vi "CRYHardware.vi"(0 "Setup in":T6={"No.VI"=0, "Category"="", "StepName"="", "Seq setup flattened"="", "Comment"="", "Steps config."=[], "Jump config"=[], "Start"=0.0, "Increment"=0.0, "Name"="Pa", "Unit"="Pa", "Y data"=1, "Y prefix"="", "Y dB ref"=1.0, "Y unit"="", "Repeat State Array"=[]} {"Repeat State Array"."Start" format="%#_5g"; "Y dB ref" format="%.1f"; "Y data" items=["dB", "Lin"]; "Start" format="%#_5g"}, 5 "Data in":T4 {"Z data" items=["dB", "Lin"]; "X data" items=["dB", "Lin"]; "Y data" items=["dB", "Lin"]; "Z dB ref" format="%.1f"; "Z axis" items=["Log", "Lin"]; "X dB ref" format="%.1f"; "X axis" items=["Log", "Lin"]; "Y axis" items=["Log", "Lin"]; "Y dB ref" format="%.1f"; "Curve"."z" format="%.2f"; "Curve"."y" format="%.2f"; "Curve"."x" format="%.2f"}, 7 "Results in":T2 {"Margin" format="%.2f"}, 9 "Seq Setup in":string, 11 "Step name":string, 12 "Hardware in":string, 13 "Calibration in":string) -> (3 "Types Out":string[](array[string]), 4 "Inserted Names Out":string[](array[string]), 6 "Data out":T4 {"Z data" items=["dB", "Lin"]; "X data" items=["dB", "Lin"]; "Y data" items=["dB", "Lin"]; "Z dB ref" format="%.1f"; "Z axis" items=["Log", "Lin"]; "X dB ref" format="%.1f"; "X axis" items=["Log", "Lin"]; "Y axis" items=["Log", "Lin"]; "Y dB ref" format="%.1f"; "Curve"."z" format="%.2f"; "Curve"."y" format="%.2f"; "Curve"."x" format="%.2f"}, 8 "Results out":T2 {"Margin" format="%.2f"}, 10 "Wave out":T1[](array[typedef]) {"Y dB ref" format="%.1f"; "Y axis" items=["Log", "Lin"]; "Y data" items=["dB", "Lin"]; "X data" items=["dB", "Lin"]})   [LabVIEW 2013]
uses:
  Typedef Control/CRYData Cluster Array.ctl
  Typedef Control/CRYData Cluster.ctl
  Typedef Control/CRYResult Cluster Array.ctl
  Typedef Control/CRYResult Cluster.ctl
  Typedef Control/CRYStep.ctl
  Typedef Control/CRYWaveform Cluster.ctl
  CRYHardware Global.vi
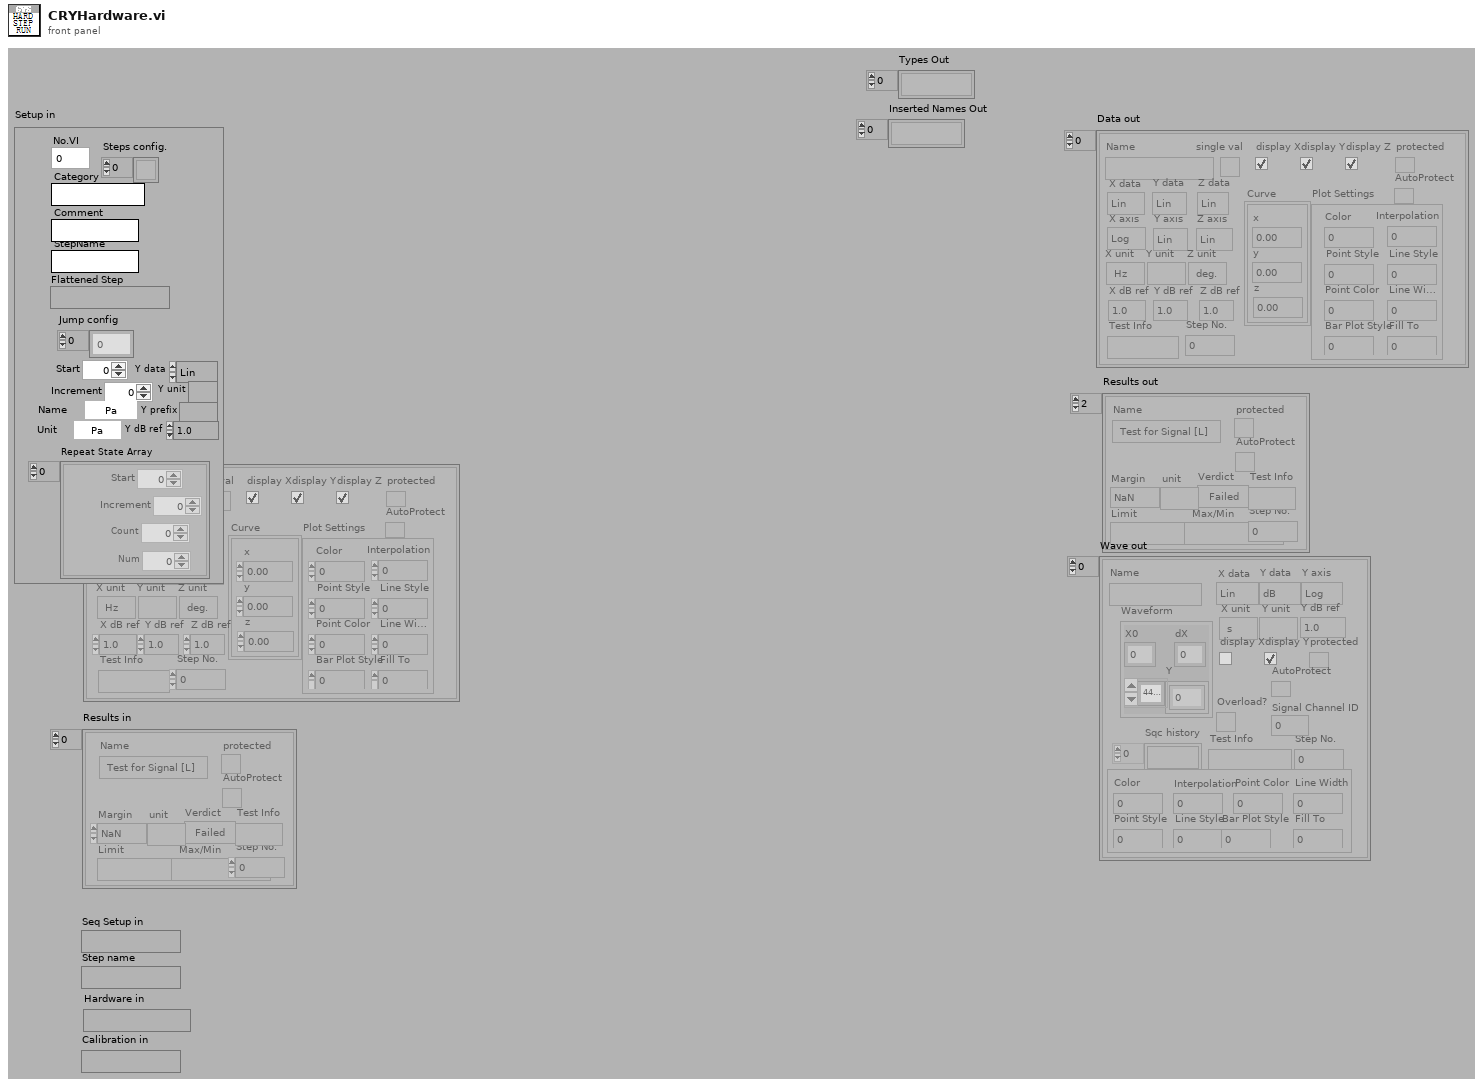
[diagram p1: front panel]
types:
  T1 = typedef "CRYWaveform Cluster.ctl" = cluster{"Waveform":cluster{"X0":dbl, "dX":dbl, "Y":sgl[]}, "X data":u16, "Y data":u16, "Y axis":u16, "X unit":string, "Y unit":string, "Y dB ref":dbl, "display Y":bool, "display X":bool, "Overload?":bool, "Test Info":string, "Step No.":i32, "Name":string, "protected":bool, "Sqc history":string[], "Signal Channel ID":i32, "Plot Settings":cluster{"Color":u32, "Interpolation":u8, "Point Style":u8, "Line Style":u8, "Point Color":u32, "Line Width":u8, "Bar Plot Style":u8, "Fill To":i16}, "AutoProtect":bool}
  T2 = typedef "CRYResult Cluster Array.ctl" = T3[]
  T3 = typedef "CRYResult Cluster.ctl" = cluster{"Name":string, "Margin":dbl, "unit":string, "Verdict":bool, "Limit":string, "Max/Min":string, "protected":bool, "Step No.":i32, "Test Info":string, "AutoProtect":bool}
  T4 = typedef "CRYData Cluster Array.ctl" = T5[]
  T5 = typedef "CRYData Cluster.ctl" = cluster{"Name":string, "Curve":cluster{"x":dbl, "y":dbl, "z":dbl}[], "X data":u16, "Y data":u16, "Z data":u16, "X axis":u16, "Y axis":u16, "Z axis":u16, "X unit":string, "Y unit":string, "Z unit":string, "X dB ref":dbl, "Y dB ref":dbl, "Z dB ref":dbl, "single val":bool, "protected":bool, "display X":bool, "display Y":bool, "display Z":bool, "Test Info":string, "Step No.":i32, "Plot Settings":cluster{"Color":u32, "Interpolation":u8, "Point Style":u8, "Line Style":u8, "Point Color":u32, "Line Width":u8, "Bar Plot Style":u8, "Fill To":i16}, "AutoProtect":bool}
  T6 = typedef "CRYStep.ctl" = cluster{"No.VI":i32, "Category":string, "StepName":string, "Seq setup flattened":string, "Comment":string, "Steps config.":bool[], "Jump config":i32[], "Start":dbl, "Increment":dbl, "Name":string, "Unit":string, "Y data":u16, "Y prefix":string, "Y dB ref":dbl, "Y unit":string, "Repeat State Array":cluster{"Start":dbl, "Increment":dbl, "Count":i32, "Num":i32}[]}
  T7 = typedef "CRY6175Hardware.ctl" = cluster{"Tab Value":u16, "Help":string, "In Channel 1":u16, "In Channel 2":u16, "In Gain 1":i32, "In Gain 2":i32, "Mic Volt":i32, "Mic Resis":i32, "Out Channel":u16, "OUT_Impedance 1":u16, "OUT_Impedance 2":u16, "IN_Channel 1 Old":u16}
  T8 = enum16{"OK", "Yes", "YesNo", "YesNoCancel", "ReplaceAppend"}
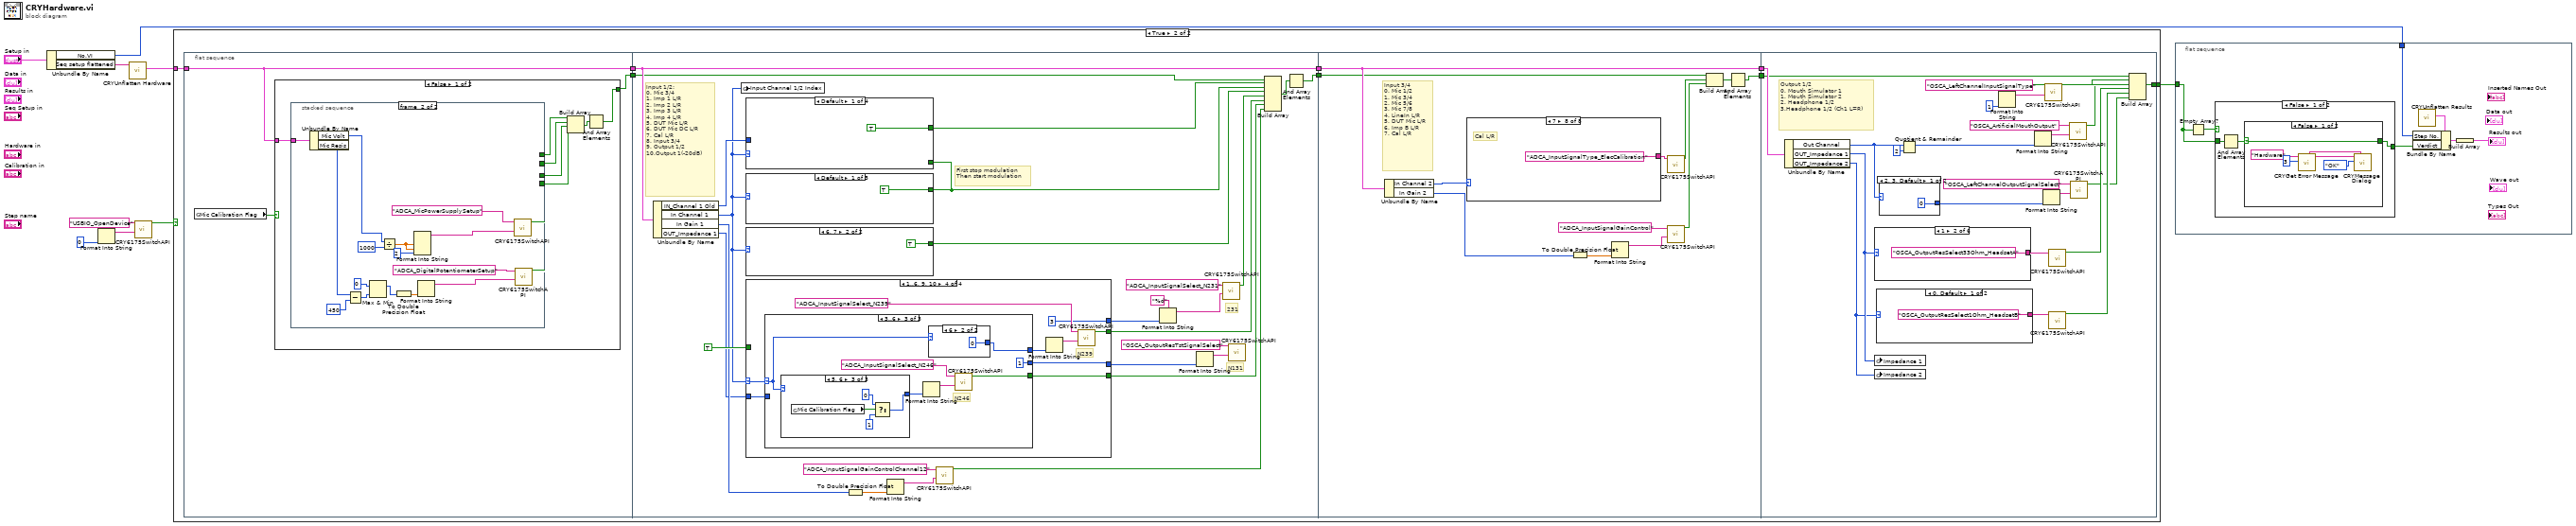
[diagram p0: block diagram]
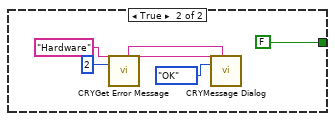
[diagram p3: hidden frame]
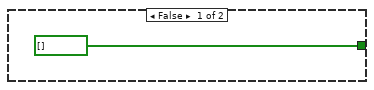
[diagram p4: hidden frame]
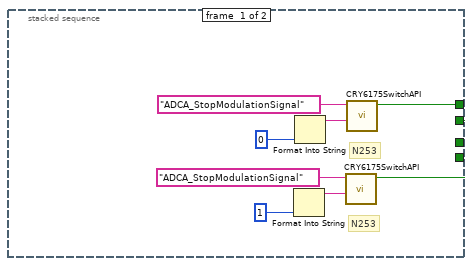
[diagram p5: hidden frame]
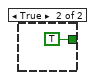
[diagram p6: hidden frame]
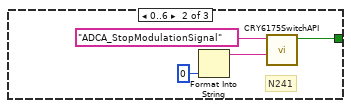
[diagram p7: hidden frame]
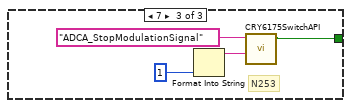
[diagram p8: hidden frame]
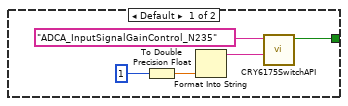
[diagram p9: hidden frame]
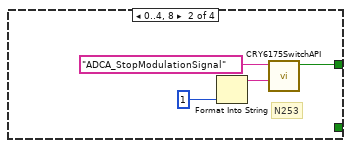
[diagram p10: hidden frame]
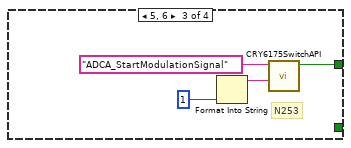
[diagram p11: hidden frame]
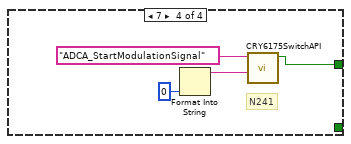
[diagram p12: hidden frame]
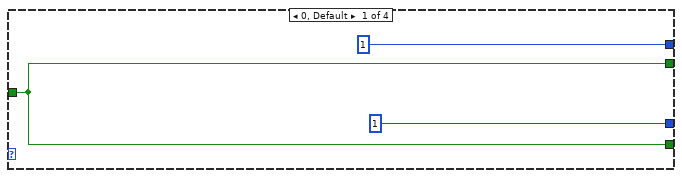
[diagram p13: hidden frame]
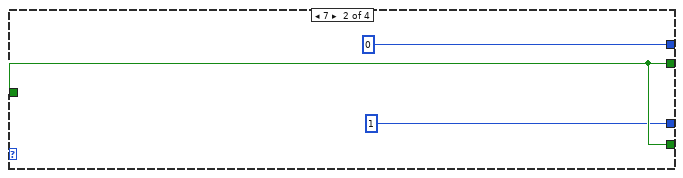
[diagram p14: hidden frame]
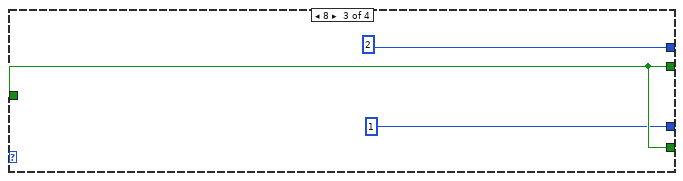
[diagram p15: hidden frame]
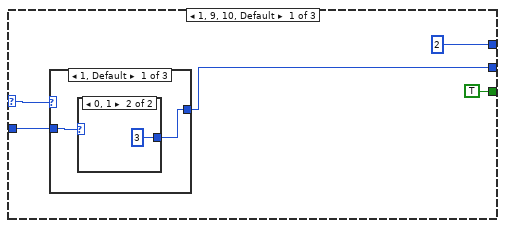
[diagram p16: hidden frame]
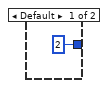
[diagram p17: hidden frame]
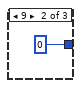
[diagram p18: hidden frame]
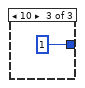
[diagram p19: hidden frame]
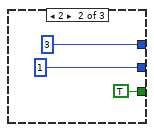
[diagram p20: hidden frame]
diagram:
  n1 = Unbundle By Name("Setup in") -> ("No.VI"=w2:i32, "Seq setup flattened"=w8:string)
  n2 = Format Into String(0) -> (resulting string=w3:string)  [unwired: 3 in, 1 out]
  n3 = call "CRYUnflatten Hardware.vi"("Unflatten Hardware#"=w8) -> ("Hardware"=w6:T7)  [unwired: 8 in, 2 out]
  n4 = call "CRY6175SwitchAPI.vi"("Parameter"=w3, "Function Name"="USBIO_OpenDevice") -> ("bResult"=w1:bool)  [unwired: 9 in]
  n5 = case shown="True" w1 {
    tunnel: w6 -> [_ w12]
    tunnel: [bool[] [] w14] -> w7
    frame False {
    }
    frame True {
      n6 = flat-sequence {
        tunnel: [w20] -> w13
        tunnel: w12 -> [w20]
        tunnel: [w21] -> w11
        tunnel: [w56] -> w18
        tunnel: [w62] -> w16
        tunnel: w13 -> [w56]
        tunnel: w11 -> [w55]
        tunnel: w18 -> [w162]
        tunnel: [w162] -> w17
        tunnel: w16 -> [w161]
        tunnel: [w157] -> w15
        tunnel: w17 -> [w198]
        tunnel: w15 -> [w192]
        tunnel: [w188] -> w14
        frame #0 {
          n7 = global read "CRYHardware Global.vi" "Mic Calibration Flag"() -> (w19:bool)
          n8 = case shown="False" w19 {
            tunnel: [w22 TRUE] -> w21
            tunnel: w20 -> [w23 _]
            frame False {
              n9 = stacked-sequence {
                tunnel: [w29 _] -> w25
                tunnel: [w30 _] -> w26
                tunnel: w23 -> [_ w39]
                tunnel: [_ w38] -> w28
                tunnel: [_ w37] -> w27
                frame #0 {
                  # "N253"
                  # "N253"
                  n10 = Format Into String(u16 1 ("input 1")) -> (resulting string=w32:string)  [unwired: 3 in, 1 out]
                  n11 = Format Into String(u16 0 ("input 1")) -> (resulting string=w35:string)  [unwired: 3 in, 1 out]
                  n12 = call "CRY6175SwitchAPI.vi"("Parameter"=w32, "Function Name"="ADCA_StopModulationSignal") -> ("bResult"=w30:bool)  [unwired: 9 in]
                  n13 = call "CRY6175SwitchAPI.vi"("Parameter"=w35, "Function Name"="ADCA_StopModulationSignal") -> ("bResult"=w29:bool)  [unwired: 9 in]
                }
                frame #1 {
                  n14 = Unbundle By Name(w39) -> ("Mic Volt"=w52:i32, "Mic Resis"=w53:i32)
                  n15 = Subtract(x=w53, y=450) -> (x-y=w49:i32)
                  n16 = Max & Min(x=0 ("y"), y=w49) -> (max(x,y)=w51:i32)  [unwired: 1 out]
                  n17 = Divide(x=w52, y=1000) -> (x/y=w44:dbl)
                  n18 = To Double Precision Float(number=w51) -> (double precision float=w41:dbl)
                  n19 = Format Into String(w44, w44, 2 ("input 3")) -> (resulting string=w42:string)  [unwired: 3 in, 1 out]
                  n20 = Format Into String(w41) -> (resulting string=w40:string)  [unwired: 3 in, 1 out]
                  n21 = call "CRY6175SwitchAPI.vi"("Parameter"=w42, "Function Name"="ADCA_MicPowerSupplySetup") -> ("bResult"=w37:bool)  [unwired: 9 in]
                  n22 = call "CRY6175SwitchAPI.vi"("Parameter"=w40, "Function Name"="ADCA_DigitalPotentiometerSetup") -> ("bResult"=w38:bool)  [unwired: 9 in]
                }
              }
              n23 = Build Array(w25, w26, w27, w28) -> (w24:bool[])
              n24 = And Array Elements(Boolean array=w24) -> (logical AND=w22:bool)
            }
            frame True {
            }
          }
        }
        frame #1 {
          # "First stop modulation\nThen start modulation"
          # "Input 1/2:\n0. Mic 3/4\n1. Imp 1 L/R\n2. Imp 2 L/R\n3. Imp 3 L/R\n4. Imp 4 L/R\n5. DUT Mic L/R\n6. DUT Mic DC L/R\n7. Cal L/R\n8. Input 3/4\n9. Output 1/2 \n10.Output 1(-20dB)"
          # "N131"
          # "231"
          n25 = Unbundle By Name(w56) -> ("IN_Channel 1 Old"=w61:u16, "In Channel 1"=w57:u16, "In Gain 1"=w60:i32, "OUT_Impedance 1"=w58:u16)
          n26 = global write "CRYHardware Global.vi" "Input Channel 1/2 Index"(w57) -> ()
          n27 = case shown="Default" w57 {
            tunnel: [TRUE ("bResult") w82 w86] -> w59
            frame Default {
            }
            frame 0..6 {
              # "N241"
              n28 = Format Into String(u16 0 ("input 1")) -> (resulting string=w85:string)  [unwired: 3 in, 1 out]
              n29 = call "CRY6175SwitchAPI.vi"("Parameter"=w85, "Function Name"="ADCA_StopModulationSignal") -> ("bResult"=w82:bool)  [unwired: 9 in]
            }
            frame 7 {
              # "N253"
              n30 = Format Into String(u16 1 ("input 1")) -> (resulting string=w88:string)  [unwired: 3 in, 1 out]
              n31 = call "CRY6175SwitchAPI.vi"("Parameter"=w88, "Function Name"="ADCA_StopModulationSignal") -> ("bResult"=w86:bool)  [unwired: 9 in]
            }
          }
          n32 = case shown="Default" w57 {
            tunnel: [TRUE ("bResult") w99 w104 w105] -> w65
            tunnel: w61 -> [_ _ _ _]
            tunnel: w59 -> [_ _ _ _]
            frame Default {
            }
            frame 0..4, 8 {
              # "N253"
              n33 = Format Into String(u16 1 ("input 1")) -> (resulting string=w98:string)  [unwired: 3 in, 1 out]
              n34 = call "CRY6175SwitchAPI.vi"("Parameter"=w98, "Function Name"="ADCA_StopModulationSignal") -> ("bResult"=w99:bool)  [unwired: 9 in]
            }
            frame 5, 6 {
              # "N253"
              n35 = Format Into String(u16 1 ("input 1")) -> (resulting string=w102:string)  [unwired: 3 in, 1 out]
              n36 = call "CRY6175SwitchAPI.vi"("Parameter"=w102, "Function Name"="ADCA_StartModulationSignal") -> ("bResult"=w104:bool)  [unwired: 9 in]
            }
            frame 7 {
              # "N241"
              n37 = Format Into String(u16 0 ("input 1")) -> (resulting string=w106:string)  [unwired: 3 in, 1 out]
              n38 = call "CRY6175SwitchAPI.vi"("Parameter"=w106, "Function Name"="ADCA_StartModulationSignal") -> ("bResult"=w105:bool)  [unwired: 9 in]
            }
          }
          n39 = case shown="6, 7" w57 {
            tunnel: [w90 TRUE ("bResult")] -> w64
            frame Default {
              n40 = To Double Precision Float(number=u16 1 ("In Channel 1")) -> (double precision float=w91:dbl)
              n41 = Format Into String(w91) -> (resulting string=w94:string)  [unwired: 3 in, 1 out]
              n42 = call "CRY6175SwitchAPI.vi"("Parameter"=w94, "Function Name"="ADCA_InputSignalGainControl_N235") -> ("bResult"=w90:bool)  [unwired: 9 in]
            }
            frame 6, 7 {
            }
          }
          n43 = case shown="1..6, 9, 10" w57 {
            selector: w57 -> [_ _ _ w126]
            tunnel: [u16 1 ("In Channel 1") u16 0 ("In Channel 1") u16 2 ("In Channel 1") u16 3 ("In Channel 1")] -> w80
            tunnel: [w110 w113 w116 w122] -> w70
            tunnel: [w110 w113 w116 w121] -> w71
            tunnel: TRUE ("bResult") -> [w110 w113 w116 _]
            tunnel: [u16 1 ("input 1") u16 1 ("input 1") u16 1 ("input 1") w119] -> w66
            tunnel: w58 -> [_ _ _ w118]
            frame 0, Default {
            }
            frame 7 {
            }
            frame 8 {
            }
            frame 1..6, 9, 10 {
              # "N239"
              n44 = case shown="3..6" w126 {
                selector: w126 -> [w129 _ w142]
                tunnel: [u16 2 ("In Channel 1") u16 3 ("In Channel 1") w141] -> w123
                tunnel: [TRUE ("bResult") TRUE ("bResult") w147] -> w122
                tunnel: [w128 u16 1 ("input 1") u16 1 ("input 1")] -> w119
                tunnel: w118 -> [w127 _ _]
                frame 1, 9, 10, Default {
                  n45 = case shown="1, Default" w129 {
                    tunnel: [w132 u16 0 ("In Channel 1") u16 1 ("In Channel 1")] -> w128
                    tunnel: w127 -> [w133 _ _]
                    frame 1, Default {
                      n46 = case shown="0, 1" w133 {
                        tunnel: [u16 2 ("In Channel 1") u16 3 ("In Channel 1")] -> w132
                        frame Default {
                        }
                        frame 0, 1 {
                        }
                      }
                    }
                    frame 9 {
                    }
                    frame 10 {
                    }
                  }
                }
                frame 2 {
                }
                frame 3..6 {
                  # "N246"
                  n47 = case shown="5, 6" w142 {
                    tunnel: [u16 2 ("In Channel 1") u16 3 ("In Channel 1") w152] -> w144
                    frame 3, Default {
                    }
                    frame 4 {
                    }
                    frame 5, 6 {
                      n48 = global read "CRYHardware Global.vi" "Mic Calibration Flag"() -> (w155:bool)
                      n49 = Select(t=u16 0 ("In Channel 1"), s=w155, f=u16 1 ("In Channel 1")) -> (s? t:f=w152:u16)
                    }
                  }
                  n50 = Format Into String(w144) -> (resulting string=w146:string)  [unwired: 3 in, 1 out]
                  n51 = case shown="6" w142 {
                    tunnel: [u16 1 ("In Channel 1") u16 0 ("In Channel 1")] -> w141
                    frame 3..5, Default {
                    }
                    frame 6 {
                    }
                  }
                  n52 = call "CRY6175SwitchAPI.vi"("Parameter"=w146, "Function Name"="ADCA_InputSignalSelect_N246") -> ("bResult"=w147:bool)  [unwired: 9 in]
                }
              }
              n53 = Format Into String(w123) -> (resulting string=w125:string)  [unwired: 3 in, 1 out]
              n54 = call "CRY6175SwitchAPI.vi"("Parameter"=w125, "Function Name"="ADCA_InputSignalSelect_N239") -> ("bResult"=w121:bool)  [unwired: 9 in]
            }
          }
          n55 = To Double Precision Float(number=w60) -> (double precision float=w79:dbl)
          n56 = Format Into String(w79) -> (resulting string=w78:string)  [unwired: 3 in, 1 out]
          n57 = call "CRY6175SwitchAPI.vi"("Parameter"=w78, "Function Name"="ADCA_InputSignalGainControlChannel12") -> ("bResult"=w69:bool)  [unwired: 9 in]
          n58 = Format Into String(format string="%d", w80) -> (resulting string=w74:string)  [unwired: 2 in, 1 out]
          n59 = Format Into String(w66) -> (resulting string=w67:string)  [unwired: 3 in, 1 out]
          n60 = call "CRY6175SwitchAPI.vi"("Parameter"=w74, "Function Name"="ADCA_InputSignalSelect_N231") -> ("bResult"=w72:bool)  [unwired: 9 in]
          n61 = call "CRY6175SwitchAPI.vi"("Parameter"=w67, "Function Name"="OSCA_OutputResTstSignalSelect") -> ()  [unwired: 9 in, 1 out]
          n62 = Build Array(w55, w65, w59, w64, w72, w71, w70, w69) -> (w63:bool[])
          n63 = And Array Elements(Boolean array=w63) -> (logical AND=w62:bool)
        }
        frame #2 {
          # "Input 3/4\n0. Mic 1/2\n1. Mic 3/4\n2. Mic 5/6\n3. Mic 7/8\n4. LineIn L/R\n5. DUT Mic L/R\n6. Imp B L/R\n7. Cal L/R"
          n64 = Unbundle By Name(w162) -> ("In Channel 2"=w163:u16, "In Gain 2"=w156:i32)
          n65 = case shown="7" w163 {
            tunnel: ["ADCA_InputSignalType_MeasurementMicrophones12" ("resulting string") "ADCA_InputSignalType_MeasurementMicrophones34" ("resulting string") "ADCA_InputSignalType_MeasurementMicrophones56" ("resulting string") "ADCA_InputSignalType_MeasurementMicrophones78" ("resulting string") "ADCA_InputSignalType_LineLR" ("resulting string") "ADCA_InputSignalType_TestedMicLR" ("resulting string") "ADCA_InputSignalType_HeadsetBImp" ("resulting string") "ADCA_InputSignalType_ElecCalibration" ("resulting string")] -> w164
            frame 0, Default {
              # "Mic 1/2"
            }
            frame 1 {
              # "Mic 3/4"
            }
            frame 2 {
              # "Mic 5/6"
            }
            frame 3 {
              # "Mic 7/8"
            }
            frame 4 {
              # "LineIn L/R"
            }
            frame 5 {
              # "DUT Mic L/R"
            }
            frame 6 {
              # "Imp B L/R"
            }
            frame 7 {
              # "Cal L/R"
            }
          }
          n66 = To Double Precision Float(number=w156) -> (double precision float=w167:dbl)
          n67 = Format Into String(w167) -> (resulting string=w166:string)  [unwired: 3 in, 1 out]
          n68 = call "CRY6175SwitchAPI.vi"("Function Name"=w164) -> ("bResult"=w160:bool)  [unwired: 10 in]
          n69 = call "CRY6175SwitchAPI.vi"("Parameter"=w166, "Function Name"="ADCA_InputSignalGainControl") -> ("bResult"=w159:bool)  [unwired: 9 in]
          n70 = Build Array(w161, w160, w159) -> (w158:bool[])
          n71 = And Array Elements(Boolean array=w158) -> (logical AND=w157:bool)
        }
        frame #3 {
          # "Output 1/2\n0. Mouth Simulator 1\n1. Mouth Simulator 2\n2. Headphone 1/2\n3.Headphone 1/2 (Ch1 L=R)"
          n72 = Unbundle By Name(w198) -> ("Out Channel"=w179:u16, "OUT_Impedance 1"=w177:u16, "OUT_Impedance 2"=w176:u16)
          n73 = case shown="1" w177 {
            tunnel: ["OSCA_OutputResSelect1Ohm_HeadsetA" ("Function Name") "OSCA_OutputResSelect33Ohm_HeadsetA" ("Function Name") "OSCA_OutputResSelect33Ohm_HeadsetA" ("Function Name") "OSCA_OutputResSelect150Ohm_HeadsetA" ("Function Name") "OSCA_OutputResSelect600Ohm_HeadsetA" ("Function Name") "OSCA_OutputResSelect750Ohm_HeadsetA" ("Function Name")] -> w197
            frame 0, Default {
            }
            frame 1 {
            }
            frame 2 {
            }
            frame 3 {
            }
            frame 4 {
            }
            frame 5 {
            }
          }
          n74 = global write "CRYHardware Global.vi" "Impedance 1"(w177) -> ()
          n75 = global write "CRYHardware Global.vi" "Impedance 2"(w176) -> ()
          n76 = case shown="0, Default" w176 {
            tunnel: ["OSCA_OutputResSelect1Ohm_HeadsetB" ("Function Name") "OSCA_OutputResSelect33Ohm_HeadsetB" ("Function Name")] -> w196
            frame 0, Default {
            }
            frame 1 {
            }
          }
          n77 = case shown="2, 3, Default" w179 {
            tunnel: [u16 0 ("input 1") u16 1 ("input 1")] -> w186
            frame 2, 3, Default {
            }
            frame 0, 1 {
            }
          }
          n78 = Quotient & Remainder(x=w179, y=u16 2) -> (x-y*floor(x/y)=w178:u16)  [unwired: 1 out]
          n79 = Format Into String(1 ("input 3")) -> (resulting string=w195:string)  [unwired: 3 in, 1 out]
          n80 = Format Into String(w178) -> (resulting string=w183:string)  [unwired: 3 in, 1 out]
          n81 = Format Into String(w186) -> (resulting string=w187:string)  [unwired: 3 in, 1 out]
          n82 = call "CRY6175SwitchAPI.vi"("Parameter"=w195, "Function Name"="OSCA_LeftChannelInputSignalType") -> ("bResult"=w191:bool)  [unwired: 9 in]
          n83 = call "CRY6175SwitchAPI.vi"("Function Name"=w197) -> ("bResult"=w190:bool)  [unwired: 10 in]
          n84 = call "CRY6175SwitchAPI.vi"("Function Name"=w196) -> ("bResult"=w189:bool)  [unwired: 10 in]
          n85 = call "CRY6175SwitchAPI.vi"("Parameter"=w183, "Function Name"="OSCA_ArtificialMouthOutput") -> ("bResult"=w181:bool)  [unwired: 9 in]
          n86 = call "CRY6175SwitchAPI.vi"("Parameter"=w187, "Function Name"="OSCA_LeftChannelOutputSignalSelect") -> ("bResult"=w185:bool)  [unwired: 9 in]
          n87 = Build Array(w192, w191, w181, w190, w189, w185) -> (w188:bool[])
        }
      }
    }
  }
  n88 = flat-sequence {
    tunnel: w7 -> [w211]
    tunnel: w2 -> [w209]
    frame #0 {
      n89 = Empty Array?(array=w211) -> (empty?=w213:bool)
      n90 = case shown="False" w213 {
        tunnel: w211 -> [w218 _]
        tunnel: [w216 FALSE ("empty?")] -> w212
        frame False {
          n91 = And Array Elements(Boolean array=w218) -> (logical AND=w217:bool)
          n92 = case shown="False" w217 {
            selector: w217 -> [w219 w225]
            tunnel: [w219 w225] -> w216
            frame False {
              n93 = call "CRYGet Error Message.vi"("Error No"=3, "Kind"="Hardware") -> ("Message"=w221:string, "Window Title"=w222:string)  [unwired: 4 in, 4 out]
              n94 = call "CRYMessage Dialog.vi"("Window Title"=w222, "YesNoCancel"=T8."OK", "Message Content"=w221) -> ()  [unwired: 7 in, 2 out]
            }
            frame True {
            }
          }
        }
        frame True {
          n95 = call "CRYGet Error Message.vi"("Error No"=2, "Kind"="Hardware") -> ("Message"=w228:string, "Window Title"=w229:string)  [unwired: 4 in, 4 out]
          n96 = call "CRYMessage Dialog.vi"("Window Title"=w229, "YesNoCancel"=T8."OK", "Message Content"=w228) -> ()  [unwired: 7 in, 2 out]
        }
      }
      n97 = call "CRYUnflatten Results.vi"() -> ("Result"=w215:T3)  [unwired: 9 in, 2 out]
      n98 = Bundle By Name(cluster=w215, "Step No."=w209, "Verdict"=w212) -> (w214:T3)
      n99 = Build Array(w214) -> (→"Results out":T3[])
    }
  }
